vi "LUnit Init.vi"(8 "error in (no error)":errorcluster, 11 "Coverage Report in":refnum<class "Coverage Report.lvclass">) -> (0 "error out":errorcluster, 3 "Coverage Report out":refnum<class "Coverage Report.lvclass">)   [LabVIEW 2020, in "Coverage Report.lvclass"]
uses:
  Coverage Report.lvclass
  Coverage Report.lvclass/Coverage Report.ctl
  <vilib>/Utility/sysdir.llb/Get System Directory.vi
  <vilib>/Utility/libraryn.llb/Create Directory Recursive.vi
  astemes-lunit/source/User Interface/Support/Paths.lvlib
  <vilib>/Astemes/LUnit/Framework/Configuration Manager/LUnit Configuration Manager.lvclass
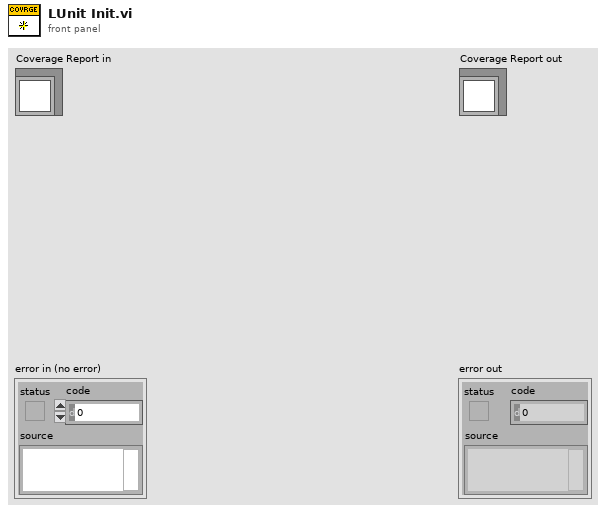
[diagram p1: front panel]
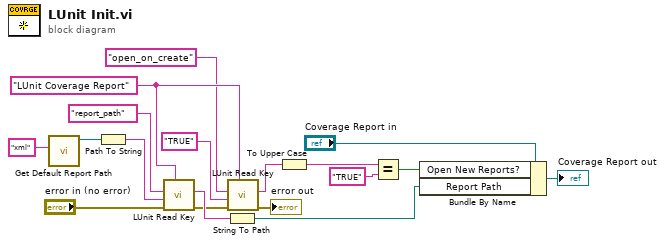
[diagram p0: block diagram]
diagram:
  w8 = "LUnit Coverage Report"
  n1 = call "Get Default Report Path.vi"("File Extension"="xml") -> ("Default Report Path"=w15:path)  [unwired: 9 in, 1 out]
  n2 = Path To String(path=w15) -> (string=w9:string)
  n3 = call <vilib>:"LUnit Read Key.vi"("section"=w8, "error in (no error)"="error in (no error)", "default value"=w9, "key"="report_path" ("Name")) -> ("error out"=w6:errorcluster, "value"=w7:string)  [unwired: 6 in]
  n4 = String To Path(string=w7) -> (path=w13:path)
  n5 = call <vilib>:"LUnit Read Key.vi"("section"=w8, "error in (no error)"=w6, "default value"="TRUE" ("y"), "key"="open_on_create" ("Name")) -> ("error out"=→"error out":errorcluster, "value"=w1:string)  [unwired: 6 in]
  n6 = To Upper Case(1:w1) -> (0:w18:string)
  n7 = Equal?(x=w18, y="TRUE") -> (x = y?=w14:bool)
  n8 = Bundle By Name(cluster="Coverage Report in", "Open New Reports?"=w14, "Report Path"=w13) -> (→"Coverage Report out":refnum<class "Coverage Report.lvclass">)
